vi "String Match Format.vi"(4 "String Format":string, 5 "String":string) -> (1 "Match format?":bool)   [LabVIEW 2019]
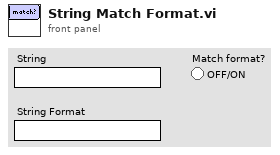
[diagram p1: front panel]
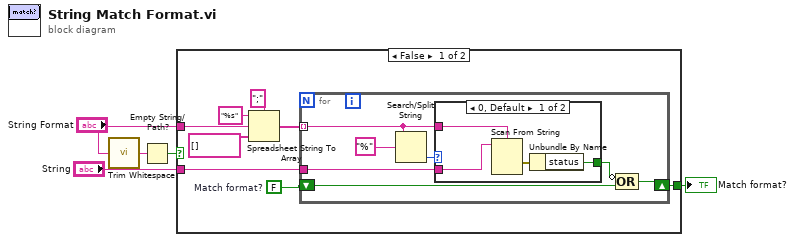
[diagram p0: block diagram]
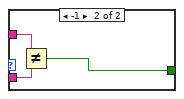
[diagram p2: hidden frame]
diagram:
  n1 = call <vilib>:"Trim Whitespace.vi"("string"="String Format") -> ("trimmed string"=w2:string)  [unwired: 1 in]
  n2 = Empty String/Path?(string/path=w2) -> (empty?=w1:bool)
  n3 = case shown="False" w1 {
    selector: w1 -> [_ w28]
    tunnel: "String" -> [w9 _]
    tunnel: [w7 w28] -> w4
    tunnel: "String Format" -> [w6 _]
    frame False {
      w8 = FALSE  # Match format?
      n4 = Spreadsheet String To Array(delimiter (Tab)=";", format string="%s", spreadsheet string=w6, array type (2D Dbl)=string[] []) -> (array=w11:string[])
      n5 = for {
        tunnel: w11 -> [w16] mode=indexing
        tunnel: w9 -> [w20]
        shift-right: [w18] -> w7
        shift-left: w8 -> [w19]
        n6 = Search/Split String(string=w16, search string/char (-)="%" ("format string")) -> (offset of match=w14:i32)  [unwired: 1 in, 2 out]
        n7 = case shown="0, Default" w14 {
          tunnel: w20 -> [w24 w26]
          tunnel: [w22 w25] -> w17
          tunnel: w16 -> [w21 w27]
          frame 0, Default {
            n8 = Scan From String(format string=w21, input string=w24) -> (error out=w23:errorcluster)  [unwired: 4 in, 2 out]
            n9 = Unbundle By Name(w23) -> ("status"=w22:bool)
          }
          frame -1 {
            n10 = Not Equal?(x=w27, y=w26) -> (x != y?=w25:bool)
          }
        }
        n11 = Compound Arithmetic op=OR(invert w17, w19) -> (w18:bool)
      }
    }
    frame True {
      # "Empty String Format: all strings match"
    }
  }
  "Match format?" <- w4
